vi "Init_XNETSesion.vi"(3 "error in (no error)":errorcluster, 4 "Model":string, 5 "interface":refnum<k21>) -> (0 "Read":refnum<k21>, 1 "error out":errorcluster, 2 "Write":refnum<k21>)   [LabVIEW 2023]
uses:
  <vilib>/xnet/xnet.llb/XNET Create Session (Frame Input Stream).vi
  <vilib>/xnet/xnet.llb/XNET Create Session (Frame Output Queued).vi
  <resource>/objmgr/xnet.rc
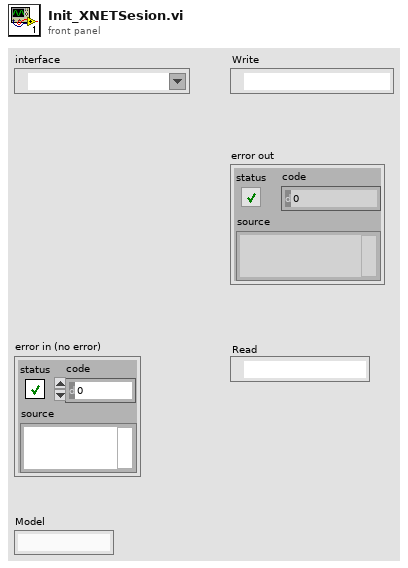
[diagram p1: front panel]
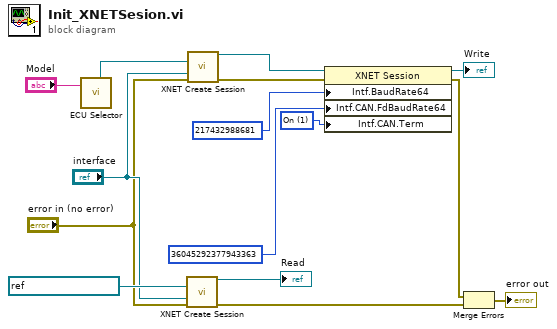
[diagram p0: block diagram]
diagram:
  w11 = u32 1 items=["Off", "On"] ("Interface:CAN:Termination")
  n1 = call "ECU Selector.vi"("Model"="Model") -> ("frame"=w6:refnum<k21>)  [unwired: 1 in, 4 out]
  n2 = call-poly <vilib>:"XNET Create Session.vi"("cluster (:memory:)"=refnum<k21> "Elatch Database", "interface"="interface", "error in (no error)"="error in (no error)") -> ("session out"=→"Read":refnum<k21>, "error out"=w3:errorcluster)  [unwired: 11 in]
  n3 = call-poly <vilib>:"XNET Create Session.vi"("frame"=w6, "interface"="interface", "error in (no error)"="error in (no error)") -> ("session out"=w10:refnum<k21>, "error out"=w15:errorcluster)  [unwired: 11 in]
  n4 = property class="XNET Session"(reference=w10, error in=w15, "Intf.BaudRate64"=u64 217432988681 ("Interface:64bit Baud Rate"), "Intf.CAN.FdBaudRate64"=u64 36045292377943363 ("Interface:CAN:64bit FD Baud Rate"), "Intf.CAN.Term"=w11) -> (reference out=→"Write":refnum<k21>, error out=w2:errorcluster)
  n5 = Merge Errors(w2, w3) -> (→"error out":errorcluster)
